vi "Convert Time To Attendance Result.vi"(8 "error in (no error)":errorcluster, 9 "上班/下班（上班）":bool, 10 "ActualTime(\"\")":string, 11 "StandardTime(\"\")":string) -> (0 "error out":errorcluster, 3 "Actual Circustance":string)   [LabVIEW 2015, in "Admin_Actor.lvlib" / "MemberAttendance.lvclass"]
uses:
  MemberAttendance.lvclass
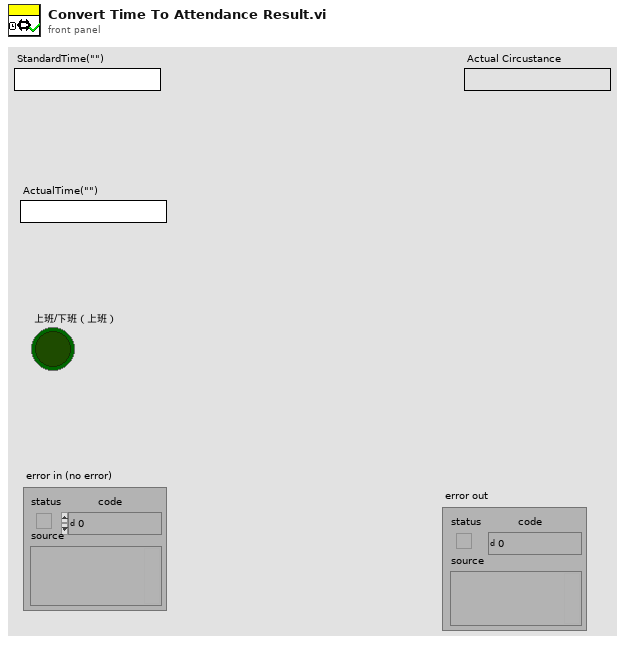
[diagram p1: front panel]
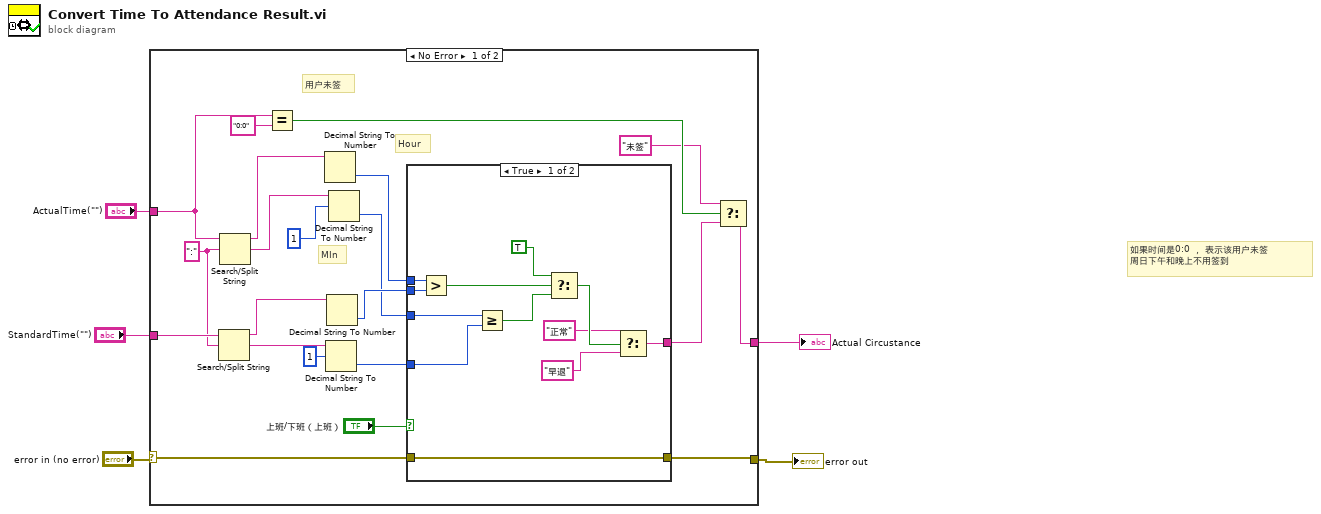
[diagram p0: block diagram]
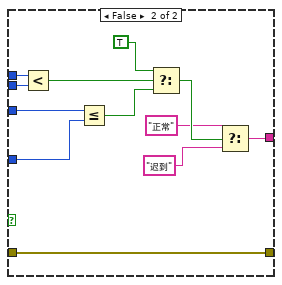
[diagram p2: hidden frame]
diagram:
  # "如果时间是0:0 ， 表示该用户未签\n周日下午和晚上不用签到"
  n1 = case shown="No Error" "error in (no error)" {
    selector: "error in (no error)" -> [w13 w51]
    tunnel: "ActualTime(\"\")" -> [w11 _]
    tunnel: "StandardTime(\"\")" -> [w25 _]
    tunnel: [w6 _] -> w3
    tunnel: [w12 w51] -> w1
    frame No Error {
      w24 = ":" ("search string/char (-)")
      # "MIn"
      # "Hour"
      # "用户未签"
      n2 = Search/Split String(string=w25, search string/char (-)=w24) -> (substring before match=w19:string, match + rest of string=w20:string)  [unwired: 1 in, 1 out]
      n3 = Search/Split String(string=w11, search string/char (-)=w24) -> (substring before match=w22:string, match + rest of string=w21:string)  [unwired: 1 in, 1 out]
      n4 = Equal?(x=w11, y="0:0") -> (x = y?=w9:bool)
      n5 = Decimal String To Number(string=w22) -> (number=w18:i32)  [unwired: 2 in, 1 out]
      n6 = Decimal String To Number(string=w20, offset=1) -> (number=w15:i32)  [unwired: 1 in, 1 out]
      n7 = Decimal String To Number(string=w19) -> (number=w17:i32)  [unwired: 2 in, 1 out]
      n8 = Decimal String To Number(string=w21, offset=1) -> (number=w14:i32)  [unwired: 1 in, 1 out]
      n9 = case shown="True" "上班/下班（上班）" {
        tunnel: w18 -> [w38 w50]
        tunnel: w17 -> [w37 w49]
        tunnel: w15 -> [w35 w47]
        tunnel: w14 -> [w36 w48]
        tunnel: [w28 w40] -> w7
        tunnel: w13 -> [w27 w39]
        tunnel: [w27 w39] -> w12
        frame True {
          n10 = Greater?(x=w38, y=w37) -> (0:w34:bool)
          n11 = Greater Or Equal?(x=w36, y=w35) -> (x >= y?=w32:bool)
          n12 = Select(t=TRUE, s=w34, f=w32) -> (s? t:f=w31:bool)
          n13 = Select(t="正常", s=w31, f="早退") -> (s? t:f=w28:string)
        }
        frame False {
          n14 = Less?(x=w50, y=w49) -> (x < y?=w46:bool)
          n15 = Less Or Equal?(x=w48, y=w47) -> (x <= y?=w44:bool)
          n16 = Select(t=TRUE, s=w46, f=w44) -> (s? t:f=w43:bool)
          n17 = Select(t="正常", s=w43, f="迟到") -> (s? t:f=w40:string)
        }
      }
      n18 = Select(t="未签", s=w9, f=w7) -> (s? t:f=w6:string)
    }
    frame Error {
    }
  }
  "Actual Circustance" <- w3
  "error out" <- w1
